vi "False Ball to Defender.vi"(4 "Campo/2":dbl, 5 "Central Position":dbl[](array[numeric]), 6 "field_width":u32, 7 "total":i32, 9 "Bola":dbl[](array[numeric]), 10 "raio da área \ndo goleiro":dbl, 11 "Our Robot in":T1={"id"=0, "function"=enum."Attacker", "x"=0.0, "y"=0.0, "orientation"=0.0, "v_tangent"=0.0, "v_normal"=0.0, "v_ang"=0.0, "kick_x"=0.0, "kick_z"=0.0, "dribble"=FALSE, "Timestamp"=timestamp(0 s since 1904-01-01), "dest_x"=0.0, "dest_y"=0.0, "dest_orientation"=0.0, "estimatives"={"est_v_tangent"=0.0, "est_v_normal"=0.0, "est_vx"=0.0, "est_vy"=0.0, "Pos Robot Est"=[]}, "dest_x_kick"=0.0, "dest_y_kick"=0.0, "Gap Coord"=[], "States"=enum."GoToTangent"}) -> (3 "Bola Falsa":dbl[](array[numeric]))   [LabVIEW 2016]
uses:
  Core/AI Robot.ctl
  Functions Enum.ctl
  AttackerStates.ctl
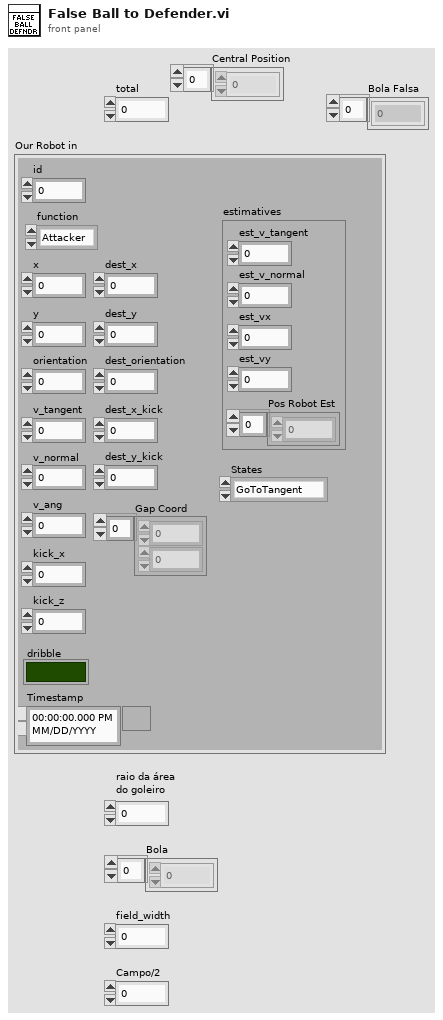
[diagram p1: front panel]
types:
  T1 = typedef "AI Robot.ctl" = cluster{"id":u32, "function":T2, "x":dbl, "y":dbl, "orientation":dbl, "v_tangent":dbl, "v_normal":dbl, "v_ang":dbl, "kick_x":dbl, "kick_z":dbl, "dribble":bool, "Timestamp":timestamp, "dest_x":dbl, "dest_y":dbl, "dest_orientation":dbl, "estimatives":cluster{"est_v_tangent":dbl, "est_v_normal":dbl, "est_vx":dbl, "est_vy":dbl, "Pos Robot Est":dbl[]}, "dest_x_kick":dbl, "dest_y_kick":dbl, "Gap Coord":dbl[], "States":T3}
  T2 = typedef "Functions Enum.ctl" = enum16{"Attacker", "Goalie", "Defender", "Striker", "Goto 0", "Dummy", "Kicker", "ZigZag"}
  T3 = typedef "AttackerStates.ctl" = enum16{"Pass", "GoToTangent", "BallGetting", "GoToKick", ""}
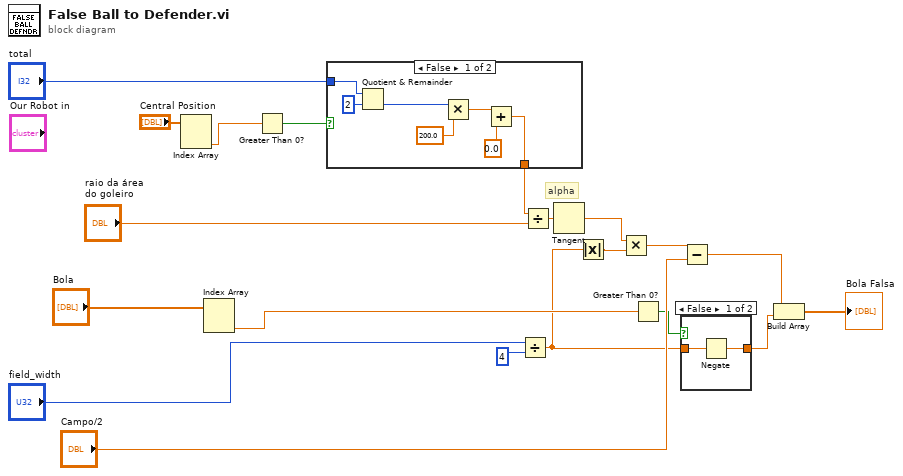
[diagram p0: block diagram]
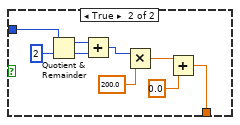
[diagram p2: hidden frame]
diagram:
  # "alpha"
  n1 = Index Array(array="Central Position") -> (element #2=w2:dbl)  [unwired: 2 in, 1 out]
  n2 = Index Array(array="Bola") -> (element #2=w20:dbl)  [unwired: 2 in, 1 out]
  n3 = Greater Than 0?(x=w2) -> (x > 0?=w12:bool)
  n4 = case shown="False" w12 {
    tunnel: [w23 w32] -> w13
    tunnel: "total" -> [w22 w31]
    frame False {
      n5 = Quotient & Remainder(x=w22, y=2) -> (floor(x/y)=w21:i32)  [unwired: 1 out]
      n6 = Multiply(x=w21, y=200.0) -> (x*y=w25:dbl)
      n7 = Add(x=w25, y=0.0) -> (x+y=w23:dbl)
    }
    frame True {
      n8 = Quotient & Remainder(x=w31, y=2) -> (x-y*floor(x/y)=w30:i32, floor(x/y)=w29:i32)
      n9 = Add(x=w30, y=w29) -> (x+y=w28:i32)
      n10 = Multiply(x=w28, y=200.0) -> (x*y=w34:dbl)
      n11 = Add(x=w34, y=0.0) -> (x+y=w32:dbl)
    }
  }
  n12 = Divide(x="field_width", y=u32 4) -> (x/y=w10:dbl)
  n13 = Divide(x=w13, y="raio da área \ndo goleiro") -> (x/y=w5:dbl)
  n14 = Tangent(1:w5) -> (0:w16:dbl)
  n15 = Absolute Value(x=w10) -> (abs(x)=w6:dbl)
  n16 = Multiply(x=w16, y=w6) -> (x*y=w7:dbl)
  n17 = Greater Than 0?(x=w20) -> (x > 0?=w9:bool)
  n18 = case shown="False" w9 {
    tunnel: w10 -> [w38 w39]
    tunnel: [w37 w39] -> w11
    frame False {
      n19 = Negate(x=w38) -> (-x=w37:dbl)
    }
    frame True {
    }
  }
  n20 = Subtract(x=w7, y="Campo/2") -> (x-y=w8:dbl)
  n21 = Build Array(w8, w11) -> (→"Bola Falsa":dbl[])
